vi "set_config_cluster.vi"(8 "error in (no error)":errorcluster, 10 "config cluster variant":variant, 11 "DataCollectionDL090215 in":refnum<class "DataCollectionDL090215.lvclass">) -> (0 "error out":errorcluster, 3 "DataCollectionDL090215 out":refnum<class "DataCollectionDL090215.lvclass">)   [LabVIEW 2010, in "DataCollectionDL090215.lvclass"]
uses:
  DataCollectionDL090215.lvclass
  DataCollectionDL090215.lvclass/DataCollectionDL090215.ctl
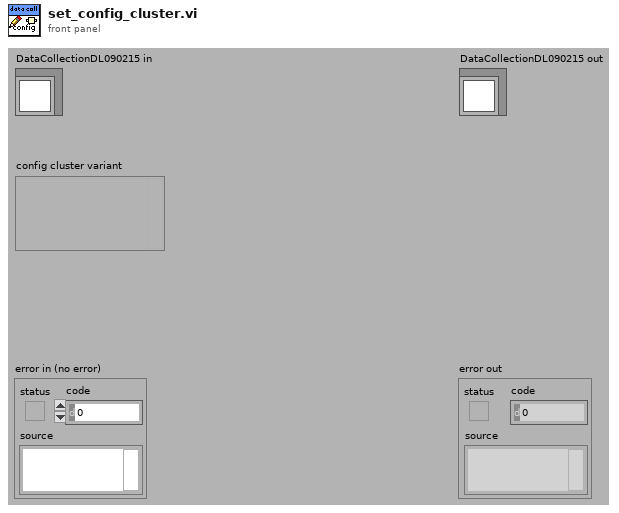
[diagram p1: front panel]
types:
  T1 = typedef "DataCollectionDL090215.lvclass/config_data_cluster.ctl" = cluster{"saving format":cluster{"channels in same file":bool, "format":T2}, "autosave default":bool, "OME default":bool}
  T2 = typedef "target_format_enum.ctl" = enum16{"don't force", "uint8", "uint16", "int16", "uint32", "int32", "single float"}
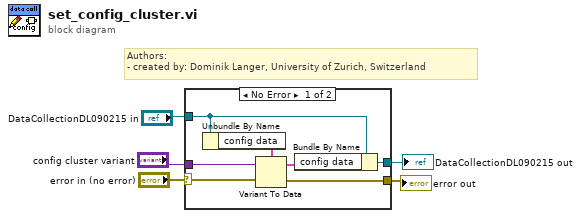
[diagram p0: block diagram]
diagram:
  # "Authors: \n- created by: Dominik Langer, University of Zurich, Switzerland"
  n1 = case shown="No Error" "error in (no error)" {
    selector: "error in (no error)" -> [w12 w13]
    tunnel: [w11 w13] -> w1
    tunnel: "DataCollectionDL090215 in" -> [w7 w14]
    tunnel: "config cluster variant" -> [w9 _]
    tunnel: [w6 w14] -> w2
    frame No Error {
      n2 = Unbundle By Name(w7) -> ("config data"=w10:T1)
      n3 = Variant To Data(error in=w12, Variant=w9, type=w10) -> (error out=w11:errorcluster, data=w8:T1)
      n4 = Bundle By Name(cluster=w7, "config data"=w8) -> (w6:refnum<class "DataCollectionDL090215.lvclass">)
    }
    frame Error {
    }
  }
  "error out" <- w1
  "DataCollectionDL090215 out" <- w2
